vi "Write Source Waveform.vi"(0 "RFFE Extended Command in":refnum<class "RFFE Extended Command.lvclass">, 5 "instrument handle":refnum<k15>, 7 "Waveform Data":u32[](array[numeric]) format="%.0x", 11 "error in (no error)":errorcluster) -> (4 "RFFE Extended Command out":refnum<class "RFFE Extended Command.lvclass">, 6 "instrument handle out":refnum<k15>, 15 "error out":errorcluster)   [LabVIEW 2018, in "MIPI RFFE API.lvlib" / "RFFE Extended Command.lvclass"]
uses:
  RFFE Extended Command.lvclass
  Command/RFFE Command.lvclass
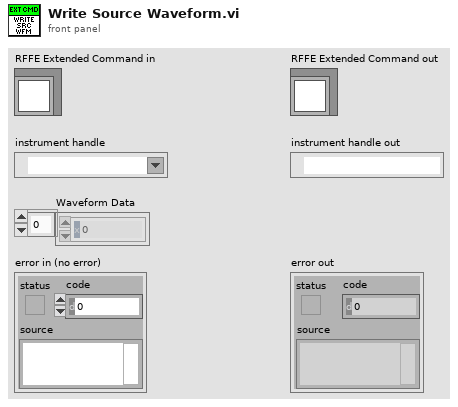
[diagram p1: front panel]
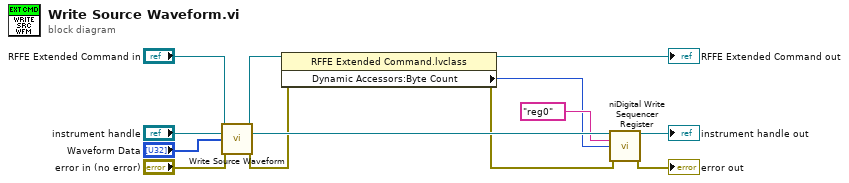
[diagram p0: block diagram]
diagram:
  n1 = call-parent "Write Source Waveform.vi"("RFFE Command in"="RFFE Extended Command in", "instrument handle"="instrument handle", "Waveform Data"="Waveform Data", "error in (no error)"="error in (no error)") -> ("RFFE Command out"=w9:refnum<class "RFFE Extended Command.lvclass">, "instrument handle out"=w7:refnum<k15>, "error out"=w4:errorcluster)  [unwired: 9 in]
  n2 = property class="RFFE Extended Command.lvclass"(reference=w9, error in=w4) -> (reference out=→"RFFE Extended Command out":refnum<class "RFFE Extended Command.lvclass">, error out=w1:errorcluster, "Dynamic Accessors:Byte Count"=w2:i32)
  n3 = call <instrlib>:"niDigital Write Sequencer Register.vi"("instrument handle"=w7, "sequencer register"="reg0", "value"=w2, "error in"=w1) -> ("instrument handle out"=→"instrument handle out":refnum<k15>, "error out"=→"error out":errorcluster)  [unwired: 10 in]
